vi "Cache-Delete.vi"(7 "Idx":i32, 8 "error in":errorcluster, 10 "Files":path[](array[path])) -> (0 "error out":errorcluster)   [LabVIEW 2016]
doc: "Go to DB->WriteStationValues action\nReturn boolean flag to show if data was saved to DB successfully\n\nWabco 2017 All right reserved\nAuthor: maciej.szupienko@wabco-auto.com"
uses:
  Cache.Action.ctl
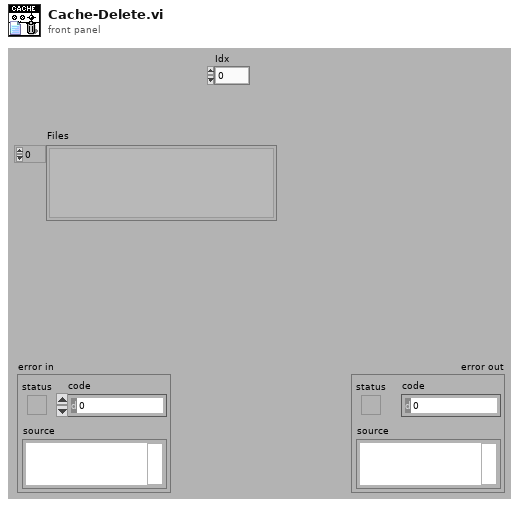
[diagram p1: front panel]
types:
  T1 = typedef "Cache.Action.ctl" = enum32{"idle", "constructor", "destructor", "--- Cache ---", "Find", "FindToExport", "Move", "Delete"}
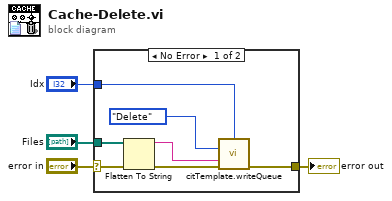
[diagram p0: block diagram]
diagram:
  n1 = case shown="No Error" "error in" {
    selector: "error in" -> [w11 w12]
    tunnel: "Idx" -> [w9 _]
    tunnel: "Files" -> [w8 _]
    tunnel: [w5 w12] -> w1
    frame No Error {
      n2 = Flatten To String(anything=w8, error in (no error)=w11) -> (data string=w7:string, error out=w6:errorcluster)  [unwired: 2 in, 1 out]
      n3 = call "citTemplate.writeQueue.vi"("instance (0)"=w9, "event in (if not connected:all statemachine with data event)"=Cache.Action."Delete" ("Action"), "data in"=w7, "error in (no error)"=w6) -> ("error out"=w5:errorcluster)  [unwired: 11 in]
    }
    frame Error {
    }
  }
  "error out" <- w1
